vi "PCO_Signal.vi"() -> (0 "PCO_Signal":T1, 1 "PCO_Signal_Raw":T2, 2 "Length":u16, 3 "Raw_Length":u16)   [LabVIEW 2019, in "SDK.lvlib" / "Structures.lvlib"]
doc: "Use this template to build a VI to use as a subVI."
uses:
  Structures.lvlib
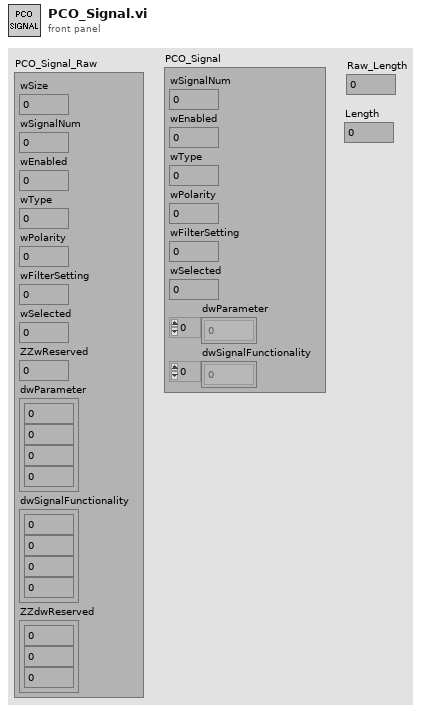
[diagram p1: front panel]
types:
  T1 = cluster{"wSignalNum":u16, "wEnabled":u16, "wType":u16, "wPolarity":u16, "wFilterSetting":u16, "wSelected":u16, "dwParameter":u32[], "dwSignalFunctionality":u32[]}
  T2 = cluster{"wSize":u16, "wSignalNum":u16, "wEnabled":u16, "wType":u16, "wPolarity":u16, "wFilterSetting":u16, "wSelected":u16, "ZZwReserved":u16, "dwParameter":cluster{u32, u32, u32, u32}, "dwSignalFunctionality":cluster{u32, u32, u32, u32}, "ZZdwReserved":cluster{u32, u32, u32}}
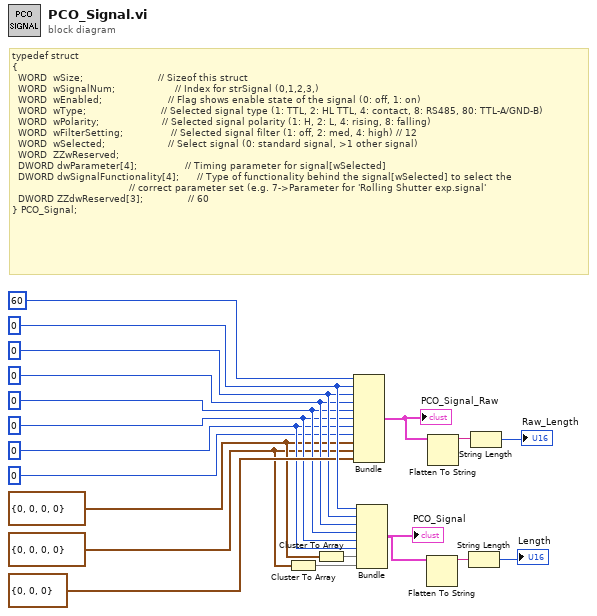
[diagram p0: block diagram]
diagram:
  w2 = cluster{u32, u32, u32, u32} {0, 0, 0, 0} ("dwSignalFunctionality")
  w4 = cluster{u32, u32, u32, u32} {0, 0, 0, 0} ("dwParameter")
  w6 = u16 0 ("wSelected")
  w7 = u16 0 ("wFilterSetting")
  w8 = u16 0 ("wPolarity")
  w9 = u16 0 ("wType")
  w10 = u16 0 ("wEnabled")
  w12 = u16 0 ("wSignalNum")
  # "typedef struct\n{\n  WORD  wSize;                         // Sizeof this struct\n  WORD  wSignalNum;                    // Index for strSignal (0,1,2,3,)\n  WORD  wEnabled;                      // Flag shows enable state of the signal (0: off, 1: on)\n  WORD  wType;                         // Selected signal type (1: TTL, 2: HL TTL, 4: contact, 8: RS485, 80: TTL-A/GND-B)\n  WORD  wPolarity;                     // Selected signal polarity (1: H, 2: L, 4: rising, 8: falling)\n  WORD  wFilterSetting;                // Selected signal filter (1: off, 2: med, 4: high) // 12\n  WORD  wSelected;                     // Select signal (0: standard signal, >1 other signal)\n  WORD  ZZwReserved;\n  DWORD dwParameter[4];                // Timing parameter for signal[wSelected]\n  DWORD dwSignalFunctionality[4];      // Type of functionality behind the signal[wSelected] to select the\n                                       // correct parameter set (e.g. 7->Parameter for 'Rolling Shutter exp.signal'\n  DWORD ZZdwReserved[3];               // 60\n} PCO_Signal;"
  n1 = Cluster To Array(cluster=w2) -> (array=w1:u32[])
  n2 = Cluster To Array(cluster=w4) -> (array=w3:u32[])
  n3 = Bundle("wSize"=u16 60, "wSignalNum"=w12, "wEnabled"=w10, "wType"=w9, "wPolarity"=w8, "wFilterSetting"=w7, "wSelected"=w6, "ZZwReserved"=u16 0, "dwParameter"=w4, "dwSignalFunctionality"=w2, "ZZdwReserved"=cluster{u32, u32, u32} {0, 0, 0}) -> (w13:T2)  [unwired: 1 in]
  "PCO_Signal_Raw" <- w13
  n4 = Bundle("wSignalNum"=w12, "wEnabled"=w10, "wType"=w9, "wPolarity"=w8, "wFilterSetting"=w7, "wSelected"=w6, "dwParameter"=w3, "dwSignalFunctionality"=w1) -> (w19:T1)  [unwired: 1 in]
  "PCO_Signal" <- w19
  n5 = Flatten To String(anything=w19) -> (data string=w18:string)  [unwired: 3 in, 2 out]
  n6 = Flatten To String(anything=w13) -> (data string=w17:string)  [unwired: 3 in, 2 out]
  n7 = String Length(string=w18) -> (length=→"Length":i32)
  n8 = String Length(string=w17) -> (length=→"Raw_Length":i32)
